vi "convertRTPCOutputBytes.vi"(8 "FullScale":dbl=24576.0, 9 "SCCM":dbl=500.0, 10 "Active Instance":u8, 11 "Setpoint":dbl) -> (3 "Bytes":u8[](array[numeric]))   [LabVIEW 2011]
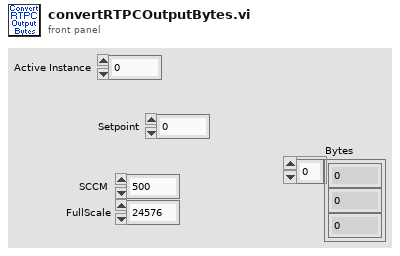
[diagram p1: front panel]
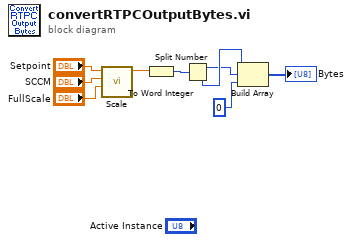
[diagram p0: block diagram]
diagram:
  n1 = call "Scale.vi"("Factor"="FullScale", "FullScale"="SCCM", "Input"="Setpoint") -> ("Output"=w9:dbl)  [unwired: 8 in]
  n2 = To Word Integer(number=w9) -> (16bit integer=w2:i16)
  n3 = Split Number(x=w2) -> (hi(x)=w4:u8, lo(x)=w5:u8)
  n4 = Build Array(w5, w4, u8 0 ("Byte 2")) -> (→"Bytes":u8[])
